vi "Andor_Acquire_old.vi"(4 "AccDoneRef":refnum<vi>, 5 "IntegTime":u32=100 caption="Integration\nTime (ms)" min=1 max=100000 step=1, 6 "Stop Acq":refnum<vi>, 7 "Accumulation":u16=1 min=1 max=256 step=1, 8 "ErrorIn(NoErr)":errorcluster, 9 "Save":bool, 10 "AndorOpQ":refnum<queue>, 11 "AndorAcqQ":refnum<queue>) -> (0 "error out":errorcluster, 1 "Delta(ms)":u32, 2 "DeltaT":u32[](array[numeric]), 3 "Data out":i32[][](array[numeric]))   [LabVIEW 2019]
uses:
  Programmes Labview/LabscanV1A/DevicesClass/InstrumentsClass/AndorSpectro/AndorAcq_States.ctl
  <userlib>/atmcd32d.llb/Error Code Enum typedef.ctl
panel:
  out "AccDone":i32
  out "imagedat":i32[](array[numeric])
  out "AcqDone":bool
  in  "Stop Acq":bool
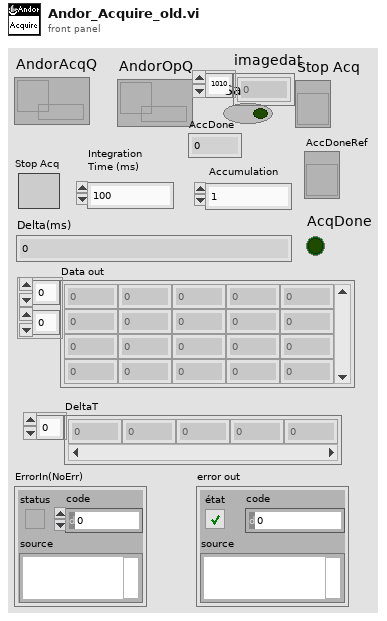
[diagram p1: front panel]
types:
  T1 = typedef "AndorAcq_States.ctl" = enum16{"Start", "Get Status", "Abort", "Error", "GetData"}
  T2 = typedef "Error Code Enum typedef.ctl" = enum32{"N/A (0)", "DRV_ERROR_CODES", "DRV_SUCCESS", "DRV_VXDNOTINSTALLED", "DRV_ERROR_SCAN", "DRV_ERROR_CHECK_SUM", "DRV_ERROR_FILELOAD", "DRV_UNKNOWN_FUNC", "DRV_ERROR_VXD_INIT", "DRV_ERROR_ADDRESS", "DRV_ERROR_PAGELOCK", "DRV_ERROR_PAGEUNLOCK", "DRV_ERROR_BOARDTEST", "DRV_ERROR_ACK", "DRV_ERROR_UP_FIFO", "DRV_ERROR_PATTERN", "N/A (16)", "DRV_ACQUISITION_ERRORS", "DRV_ACQ_BUFFER", "DRV_ACQ_DOWNFIFO_FULL", "DRV_PROC_UNKONWN_INSTRUCTION", "DRV_ILLEGAL_OP_CODE", "DRV_KINETIC_TIME_NOT_MET", "DRV_ACCUM_TIME_NOT_MET", "DRV_NO_NEW_DATA", "N/A (25)", "DRV_SPOOLERROR", "N/A (27)", "N/A (28)", "N/A (29)", "N/A (30)", "N/A (31)", "N/A (32)", "DRV_TEMPERATURE_CODES", "DRV_TEMPERATURE_OFF", "DRV_TEMPERATURE_NOT_STABILIZED", "DRV_TEMPERATURE_STABILIZED", "DRV_TEMPERATURE_NOT_REACHED", "DRV_TEMPERATURE_OUT_RANGE", "DRV_TEMPERATURE_NOT_SUPPORTED", "DRV_TEMPERATURE_DRIFT", "N/A (41)", "N/A (42)", "N/A (43)", "N/A (44)", "N/A (45)", "N/A (46)", "N/A (47)", "N/A (48)", "DRV_GENERAL_ERRORS", "DRV_INVALID_AUX", "DRV_COF_NOTLOADED", "DRV_FPGAPROG", "DRV_FLEXERROR", "DRV_GPIBERROR", "N/A (55)", "N/A (56)", "N/A (57)", "N/A (58)", "N/A (59)", "N/A (60)", "N/A (61)", "N/A (62)", "N/A (63)", "DRV_DATATYPE", "DRV_DRIVER_ERRORS", "DRV_P1INVALID", "DRV_P2INVALID", "DRV_P3INVALID", "DRV_P4INVALID", "DRV_INIERROR", "DRV_COFERROR", "DRV_ACQUIRING", "DRV_IDLE", "DRV_TEMPCYCLE", "DRV_NOT_INITIALIZED", "DRV_P5INVALID", "DRV_P6INVALID", "DRV_INVALID_MODE", "DRV_INVALID_FILTER", "DRV_I2CERRORS", "DRV_I2CDEVNOTFOUND", "DRV_I2CTIMEOUT", "DRV_P7INVALID", "N/A (84)", "N/A (85)", "N/A (86)", "N/A (87)", "N/A (88)", "N/A (89)", "DRV_IOCERROR", "DRV_VRMVERSIONERROR"}
  T3 = cluster{"Message":string, "Data":variant, "Code":i32}
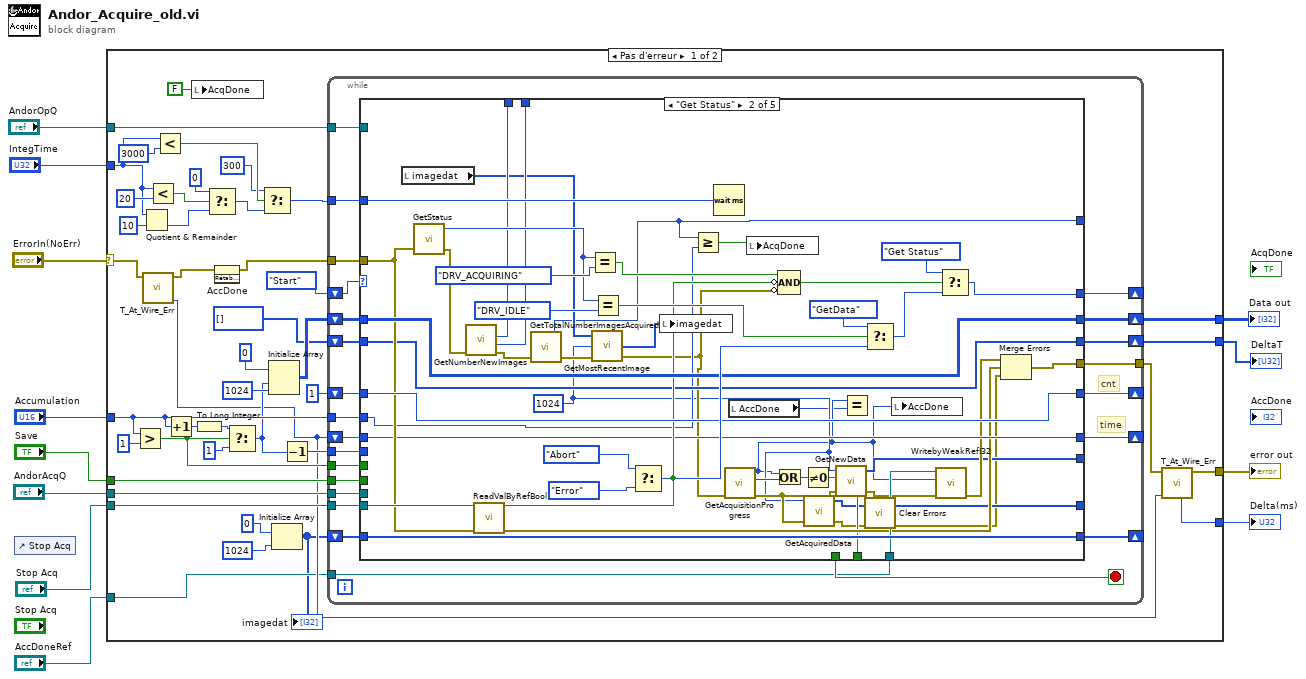
[diagram p0: block diagram]
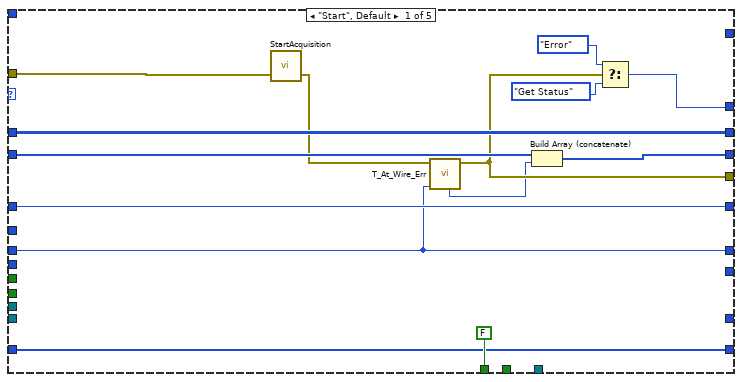
[diagram p2: hidden frame]
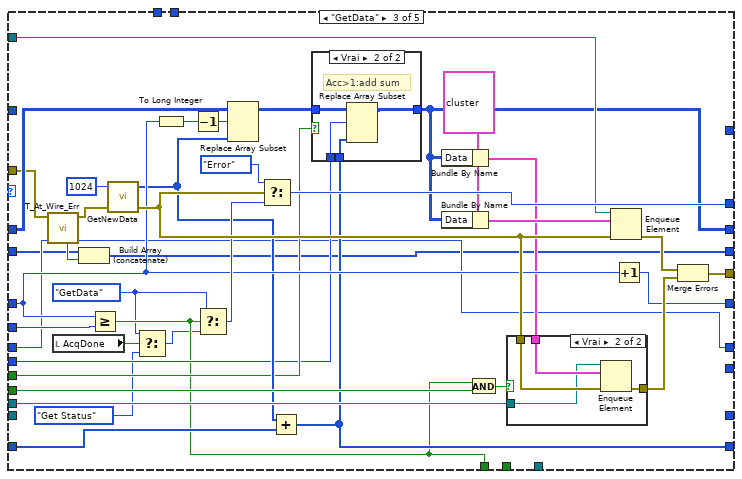
[diagram p3: hidden frame]
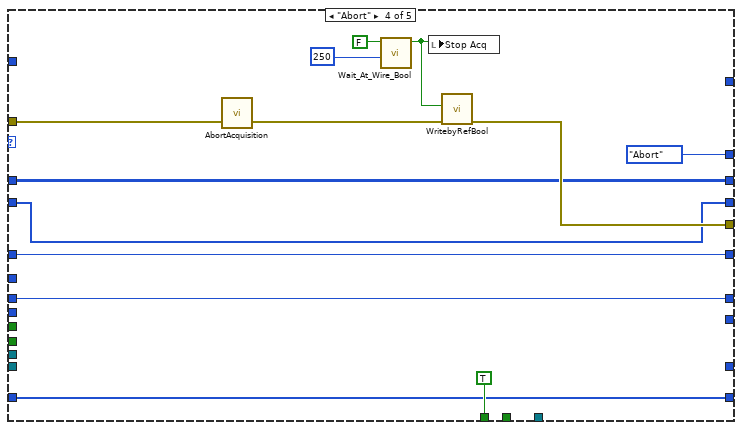
[diagram p6: hidden frame]
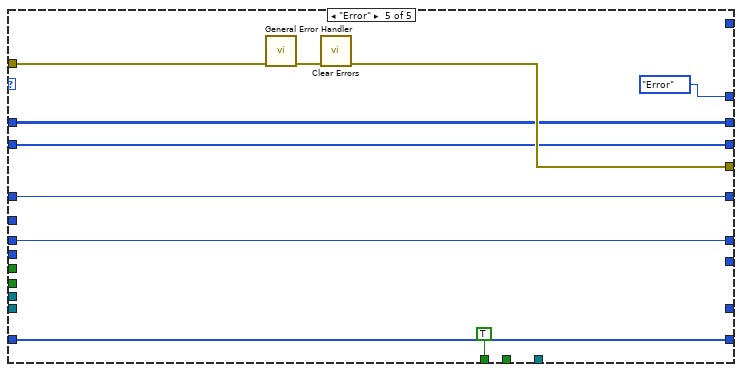
[diagram p7: hidden frame]
diagram:
  n1 = control-ref of="Stop Acq"() -> ()  [unwired: 1 out]
  n2 = case shown="Pas d'erreur" "ErrorIn(NoErr)" {
    selector: "ErrorIn(NoErr)" -> [w28 w216]
    tunnel: [w26 w216] -> w11
    tunnel: "AndorAcqQ" -> [w54 _]
    tunnel: "AndorOpQ" -> [w53 _]
    tunnel: "Save" -> [w52 _]
    tunnel: "Accumulation" -> [w40 _]
    tunnel: "Stop Acq" -> [w50 _]
    tunnel: "IntegTime" -> [w17 _]
    tunnel: [w43 _] -> w4
    tunnel: [w29 _] -> w3
    tunnel: [w24 _] -> w2
    tunnel: "AccDoneRef" -> [w23 _]
    frame No Error {
      n3 = Greater?(x=w40, y=u16 1) -> (0:w34:bool)
      n4 = Quotient & Remainder(x=w17, y=u32 10) -> (floor(x/y)=w48:u32)  [unwired: 1 out]
      n5 = call <userlib>:"T_At_Wire_Err.vi"("error in (no error)"=w28) -> ("Clock(ms)"=w25:u32, "error out"=w20:errorcluster)  [unwired: 8 in, 1 out]
      n6 = Less?(x=w17, y=u32 20 ("limite supérieure")) -> (x < y?=w31:bool)
      n7 = Less?(x=w17, y=u32 3000 ("limite supérieure")) -> (x < y?=w16:bool)
      n8 = Increment(x=w40) -> (x+1=w39:u16)
      n9 = local write "AcqDone"(FALSE ("AcqDone")) -> ()
      n10 = To Long Integer(number=w39) -> (32bit integer=w38:i32)
      n11 = Select(t=u32 0 ("cas vrai"), s=w31, f=w48) -> (s? t:f=w15:u32)
      n12 = invoke on="AccDone" class="NumNb (strict)" method="RétablirValParDéfaut"(error in=w20) -> (error out=w19:errorcluster)  [unwired: 2 in, 2 out]
      n13 = Select(t=w38, s=w34, f=1 ("y")) -> (s? t:f=w35:i32)
      n14 = Select(t=u32 300 ("cas vrai"), s=w16, f=w15) -> (s? t:f=w13:u32)
      n15 = Initialize Array(0 ("élément"), w35, 1024 ("taille de la dimension")) -> (w44:i32[][])
      n16 = Initialize Array(0 ("élément"), 1024 ("taille de la dimension")) -> (w21:i32[])
      "imagedat" <- w21
      n17 = Decrement(x=w35) -> (x-1=w33:i32)
      n18 = while {
        tunnel: [w79] -> w27
        tunnel: w19 -> [w77]
        shift-right: [w76] -> _
        shift-left: AndorAcq_States."Start" ("AndorAcqSt") -> [w78]
        tunnel: w53 -> [w74]
        tunnel: w54 -> [w73]
        tunnel: w52 -> [w72]
        tunnel: w40 -> [w71]
        shift-right: [w69] -> _
        shift-left: u16 1 -> [w70]
        tunnel: w50 -> [w68]
        tunnel: w13 -> [w67]
        shift-right: [w65] -> w43
        shift-left: w44 -> [w66]
        shift-right: [w63] -> _
        shift-left: w21 -> [w64]
        tunnel: w33 -> [w62]
        tunnel: w34 -> [w61]
        shift-right: [w57] -> _
        shift-left: w25 -> [w60]
        shift-right: [w59] -> w29
        shift-left: u32[] [] -> [w58]
        tunnel: w23 -> [w56]
        stop <- w75 stop-if-true
        # "cnt"
        # "time"
        n19 = case shown="\"Get Status\"" w78 {
          tunnel: [w83 w123 w177 w198 w211] -> w79
          tunnel: w77 -> [w86 w124 w158 w205 w215]
          tunnel: [w91 w140 w182 AndorAcq_States."Abort" ("AndorAcqSt") AndorAcq_States."Error" ("AndorAcqSt")] -> w76
          tunnel: [FALSE _ w149 TRUE TRUE] -> w75
          tunnel: w74 -> [_ _ w154 _ _]
          tunnel: w73 -> [_ _ w180 _ _]
          tunnel: w72 -> [_ _ w175 _ _]
          tunnel: w71 -> [_ w114 w161 _ _]
          tunnel: w70 -> [w89 w133 w170 w197 w210]
          tunnel: [w89 w133 w172 w197 w210] -> w69
          tunnel: w68 -> [_ w126 _ _ _]
          tunnel: w67 -> [_ w128 _ _ _]
          tunnel: w66 -> [w88 w127 w171 w196 w209]
          tunnel: [w88 w127 w144 w196 w209] -> w65
          tunnel: w64 -> [w87 w122 w164 w195 w208]
          tunnel: [w87 w122 w162 w195 w208] -> w63
          tunnel: w62 -> [_ _ w159 _ _]
          tunnel: w61 -> [_ _ w160 _ _]
          tunnel: [w82 w121 w155 w194 w207] -> w57
          tunnel: w60 -> [w82 w121 w156 w194 w207]
          tunnel: [w81 w120 w152 w193 w206] -> w59
          tunnel: w58 -> [w85 w120 w151 w193 w206]
          tunnel: w56 -> [_ w119 _ _ _]
          tunnel: [_ w103 _ _ _] -> _
          tunnel: [_ w113 _ _ _] -> _
          tunnel: [_ w109 _ _ _] -> _
          tunnel: [_ w108 _ _ _] -> _
          tunnel: [_ w102 _ _ _] -> _
          tunnel: [_ w98 _ _ _] -> _
          frame "Start", Default {
            n20 = call <userlib>:"StartAcquisition.vi"("error in (no error)"=w86) -> ("error out"=w84:errorcluster)  [unwired: 1 in, 1 out]
            n21 = call <userlib>:"T_At_Wire_Err.vi"("InitClock(ms)"=w82, "error in (no error)"=w84) -> ("error out"=w83:errorcluster, "Delta(ms)"=w80:u32)  [unwired: 7 in, 1 out]
            n22 = Build Array (concatenate)(w85, w80) -> (w81:u32[])
            n23 = Select(t=AndorAcq_States."Error" ("AndorAcqSt"), s=w83, f=AndorAcq_States."Get Status" ("AndorAcqSt")) -> (s? t:f=w91:T1)
          }
          frame "Get Status" {
            w99 = 1024 ("size")
            n24 = local read "imagedat"() -> (w106:i32[])
            n25 = call <userlib>:"GetStatus.vi"("error in (no error)"=w124) -> ("error out"=w111:errorcluster, "status"=w138:T2)  [unwired: 2 in, 1 out]
            n26 = call <userlib>:"GetNumberNewImages.vi"("error in (no error)"=w111) -> ("error out"=w110:errorcluster, "last"=w109:i32, "first"=w108:u32)  [unwired: 3 in, 1 out]
            n27 = call <userlib>:"ReadValByRefBool.vi"("Control Ref"=w126, "error in"=w124) -> ("Valeur"=w125:bool, "error out"=w117:errorcluster)  [unwired: 12 in]
            n28 = call <userlib>:"GetTotalNumberImagesAcquired.vi"("error in (no error)"=w110) -> ("error out"=w107:errorcluster, "index"=w103:i32)  [unwired: 2 in, 1 out]
            n29 = Equal?(x=w138, y=Error_Code_Enum_typedef."DRV_ACQUIRING" ("status")) -> (x = y?=w141:bool)
            n30 = call <userlib>:"GetMostRecentImage.vi"("error in (no error)"=w107, "size"=w99, "array"=w106) -> ("error out"=w104:errorcluster, "array"=w105:i32[])  [unwired: 1 out]
            n31 = Equal?(x=w138, y=Error_Code_Enum_typedef."DRV_IDLE" ("status")) -> (x = y?=w136:bool)
            n32 = Select(t=AndorAcq_States."Abort" ("AndorAcqSt"), s=w125, f=AndorAcq_States."Error" ("AndorAcqSt")) -> (s? t:f=w135:T1)
            n33 = local write "imagedat"(w105) -> ()
            n34 = Greater Or Equal?(x=w103, y=w114) -> (x >= y?=w112:bool)
            n35 = Wait (ms)(milliseconds to wait=w128) -> ()  [unwired: 1 out]
            n36 = call <userlib>:"GetAcquisitionProgress.vi"("error in (no error)"=w104) -> ("error out"=w100:errorcluster, "series"=w116:i32, "accum"=w95:i32)  [unwired: 3 in, 1 out]
            n37 = local read "AccDone"() -> (w94:i32)
            n38 = local write "AcqDone"(w112) -> ()
            n39 = Or(x=w95, y=w116) -> (x .or. y?=w115:i32)
            n40 = Compound Arithmetic op=AND ("Opérateur arithmétique")(w141, invert w125, invert w104) -> (w139:bool)
            n41 = Not Equal To 0?(x=w115) -> (x != 0?=w113:bool)
            n42 = call <userlib>:"GetAcquiredData.vi"("error in (no error)"=w100, "size"=w99) -> ("error out"=w97:errorcluster, "array"=w98:i32[])  [unwired: 1 in, 1 out]
            n43 = call <userlib>:"GetNewData.vi"("error in (no error)"=w100, "size"=w99) -> ("error out"=w101:errorcluster, "array"=w102:i32[])  [unwired: 1 in, 1 out]
            n44 = Equal?(x=w95, y=w94) -> ()  [unwired: 1 out]
            n45 = Select(t=AndorAcq_States."GetData" ("AndorAcqSt"), s=w136, f=w135) -> (s? t:f=w134:T1)
            n46 = call <vilib>:"Clear Errors.vi"("error in (no error)"=w97) -> ("error out"=w96:errorcluster)  [unwired: 5 in, 1 out]
            n47 = local write "AccDone"(w95) -> ()
            n48 = call <userlib>:"WritebyWeakRefI32.vi"("error in"=w101, "Valeur"=w95, "Control Ref"=w119) -> ("error out"=w118:errorcluster)  [unwired: 8 in]
            n49 = Select(t=AndorAcq_States."Get Status" ("AndorAcqSt"), s=w139, f=w134) -> (s? t:f=w140:T1)
            n50 = Merge Errors(w118, w117, w96) -> (w123:errorcluster)
          }
          frame "GetData" {
            w146 = AndorAcq_States."GetData" ("AndorAcqSt")
            w167 = T3 {"Message"="PlotSgl", "Data"=variant, "Code"=1}
            n51 = call <userlib>:"T_At_Wire_Err.vi"("InitClock(ms)"=w156, "error in (no error)"=w158) -> ("Clock(ms)"=w155:u32, "error out"=w157:errorcluster, "Delta(ms)"=w153:u32)  [unwired: 7 in]
            n52 = local read "AcqDone"() -> (w148:bool)
            n53 = Build Array (concatenate)(w151, w153) -> (w152:u32[])
            n54 = Greater Or Equal?(x=w170, y=w161) -> (x >= y?=w149:bool)
            n55 = call <userlib>:"GetNewData.vi"("error in (no error)"=w157, "size"=u32 1024) -> ("error out"=w178:errorcluster, "array"=w165:i32[])  [unwired: 1 in, 1 out]
            n56 = Select(t=w146, s=w148, f=AndorAcq_States."Get Status" ("AndorAcqSt")) -> (s? t:f=w145:T1)
            n57 = To Long Integer(number=w170) -> (32bit integer=w168:i32)
            n58 = Decrement(x=w168) -> (x-1=w169:i32)
            n59 = Select(t=w146, s=w149, f=w145) -> (s? t:f=w173:T1)
            n60 = Replace Array Subset(array=w171, new element=w165, index (row)=w169) -> (w163:i32[][])  [unwired: 1 in]
            n61 = Select(t=AndorAcq_States."Error" ("AndorAcqSt"), s=w178, f=w173) -> (s? t:f=w182:T1)
            n62 = Add(x=w165, y=w164) -> (x+y=w162:i32[])
            n63 = case shown="Vrai" w160 {
              tunnel: w163 -> [w183 w187]
              tunnel: w162 -> [_ w186]
              tunnel: w159 -> [_ w185]
              tunnel: [w183 w184] -> w144
              frame False {
              }
              frame True {
                # "Acc>1:add sum"
                n64 = Replace Array Subset(array=w187, new element=w186, index (row)=w185) -> (w184:i32[][])  [unwired: 1 in]
              }
            }
            n65 = Bundle By Name(cluster=w167, "Data"=w144) -> (w166:T3)
            n66 = Bundle By Name(cluster=w167, "Data"=w144) -> (w179:T3)
            n67 = And(x=w149, y=w175) -> (x .and. y?=w150:bool)
            n68 = case shown="Vrai" w150 {
              tunnel: w180 -> [_ w189]
              tunnel: w166 -> [_ w192]
              tunnel: w178 -> [w188 w191]
              tunnel: [w188 w190] -> w176
              frame False {
              }
              frame True {
                n69 = Enqueue Element(queue=w189, element=w192, error in (no error)=w191) -> (error out=w190:errorcluster)  [unwired: 1 in, 2 out]
              }
            }
            n70 = Enqueue Element(queue=w154, element=w179, error in (no error)=w178) -> (error out=w181:errorcluster)  [unwired: 1 in, 2 out]
            n71 = Increment(x=w170) -> (x+1=w172:u16)
            n72 = Merge Errors(w181, w176) -> (w177:errorcluster)
          }
          frame "Abort" {
            n73 = call <userlib>:"AbortAcquisition.vi"("error in (no error)"=w205) -> ("error out"=w200:errorcluster)  [unwired: 1 in, 1 out]
            n74 = call <userlib>:"Wait_At_Wire_Bool.vi"("Wait (ms)"=u32 250, "error in (no error)"=FALSE) -> ("error out"=w199:bool)  [unwired: 7 in, 2 out]
            n75 = local write "Stop Acq"(w199) -> ()
            n76 = call <userlib>:"WritebyRefBool.vi"("error in"=w200, "Valeur"=w199) -> ("error out"=w198:errorcluster)  [unwired: 9 in]
          }
          frame "Error" {
            n77 = call <vilib>:"General Error Handler.vi"("error in (no error)"=w215) -> ("error out"=w214:errorcluster)  [unwired: 10 in, 4 out]
            n78 = call <vilib>:"Clear Errors.vi"("error in (no error)"=w214) -> ("error out"=w211:errorcluster)  [unwired: 5 in, 1 out]
          }
        }
      }
      n79 = call <userlib>:"T_At_Wire_Err.vi"("InitClock(ms)"=w25, "error in (no error)"=w27) -> ("error out"=w26:errorcluster, "Delta(ms)"=w24:u32)  [unwired: 7 in, 1 out]
    }
    frame Error {
    }
  }
  "error out" <- w11
  "Data out" <- w4
  "DeltaT" <- w3
  "Delta(ms)" <- w2
